vi "Write lockin.vi"(8 "error in (no error)":errorcluster, 10 "lockin":T4, 11 "lockin in":refnum<class "lockin.lvclass">) -> (0 "error out":errorcluster, 3 "lockin out":refnum<class "lockin.lvclass">)   [LabVIEW 2016, in "lockin.lvclass"]
uses:
  lockin.lvclass
  Typedefs/lockin_configuration.ctl
  Typedefs/lockin_input_signals.ctl
  Typedefs/lockin_results.ctl
  lockin.lvclass/lockin.ctl
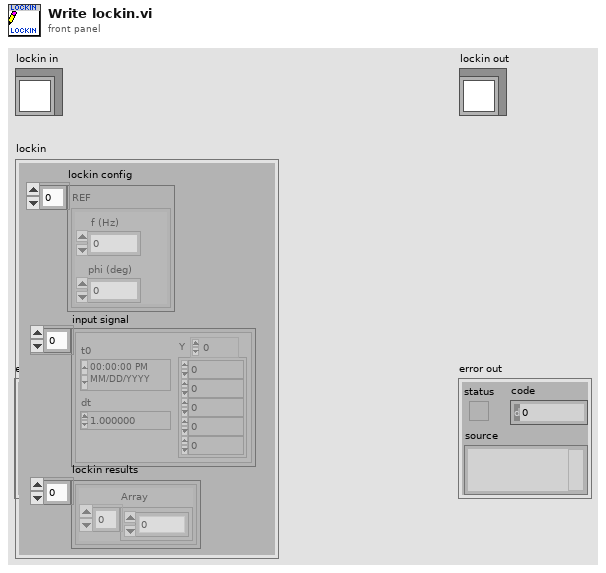
[diagram p1: front panel]
types:
  T1 = typedef "lockin.lvclass/lockin_configuration.ctl" = cluster{" f (Hz)":dbl, "phi (deg)":dbl}[]
  T2 = typedef "lockin.lvclass/lockin_input_signals.ctl" = waveform(dbl)[]
  T3 = typedef "lockin.lvclass/lockin_results.ctl" = cluster{"Array":dbl[]}[]
  T4 = cluster{"lockin config":T1, "input signal":T2, "lockin results":T3}
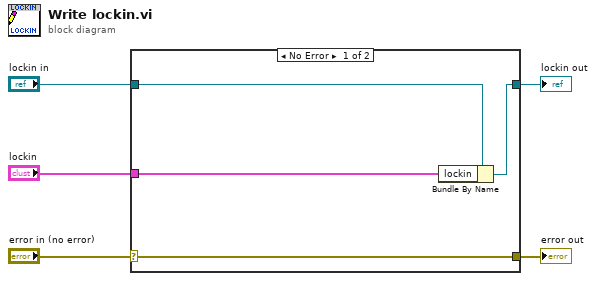
[diagram p0: block diagram]
diagram:
  n1 = case shown="No Error" "error in (no error)" {
    selector: "error in (no error)" -> [w9 w10]
    tunnel: [w9 w10] -> w4
    tunnel: [w7 w11] -> w2
    tunnel: "lockin in" -> [w8 w11]
    tunnel: "lockin" -> [w6 _]
    frame No Error {
      n2 = Bundle By Name(cluster=w8, "lockin"=w6) -> (w7:refnum<class "lockin.lvclass">)
    }
    frame Error {
    }
  }
  "error out" <- w4
  "lockin out" <- w2
